vi "Update Chart Axis Names.vi"(0 "Chart":refnum<vi>, 5 "Y Axis Names":string[](array[string]), 7 "X Axis Name":string) -> ()   [LabVIEW 2019]
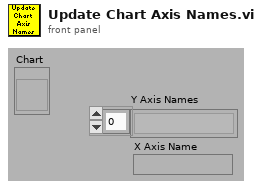
[diagram p1: front panel]
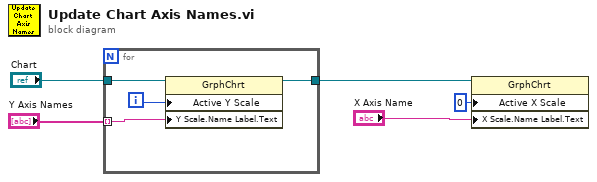
[diagram p0: block diagram]
diagram:
  n1 = for {
    tunnel: "Chart" -> [w9]
    tunnel: "Y Axis Names" -> [w7] mode=indexing
    tunnel: [w6] -> w3
    i -> [w8]
    n2 = property class="GrphChrt"(reference=w9, "Active Y Scale"=w8, "Y Scale.Name Label.Text"=w7) -> (reference out=w6:refnum<vi>)  [unwired: 1 in, 1 out]
  }
  n3 = property on="Property Node" class="GrphChrt"(reference=w3, "Active X Scale"=0, "X Scale.Name Label.Text"="X Axis Name") -> ()  [unwired: 1 in, 2 out]
